vi "Get Tweets New.vi"(8 "error in":errorcluster, 9 "Tweets to Read (10)":i32=10 min=0 max=200 step=1, 10 "Screen Name (Empty)":string, 11 "Twitter Handle In":T2={"OAuth Credentials"={"Consumer Key"="", "Signature Method"=enum."HMAC-SHA1", "Token"="", "Version"="", "Token Secret"="", "Consumer Secret"=""}, "since ID"="", "max ID"="", "Screen Name"=""}) -> (0 "error out":errorcluster, 1 "Actual Num of Tweets Read":i32, 2 "New Tweets Read":T1[](array[typedef]), 3 "Twitter Handle Out":T2={"OAuth Credentials"={"Consumer Key"="", "Signature Method"=enum."HMAC-SHA1", "Token"="", "Version"="", "Token Secret"="", "Consumer Secret"=""}, "since ID"="", "max ID"="", "Screen Name"=""}, 5 "Time Stamp of Newest Tweet":timestamp)   [LabVIEW 2011, in "i3-twitter.lvlib"]
doc: "Get new tweets for the screen name. If no screen name is provided, tweets for the authenticating user are returned."
uses:
  i3-twitter.lvlib
  Controls/Twitter Handle.ctl
  i3-oauth/Controls/OAuth Credentials.ctl
  i3-oauth/Controls/Signature Method.ctl
  Controls/Tweet.ctl
  i3-oauth/Controls/HTTP Method.ctl
  i3-oauth/i3-oauth.lvlib
  <vilib>/httpClient/LabVIEWHTTPClient.lvlib
  i3-json/i3-json.lvlib
panel:
  out "headers":string
  out "body":string
  out "Full URL":string
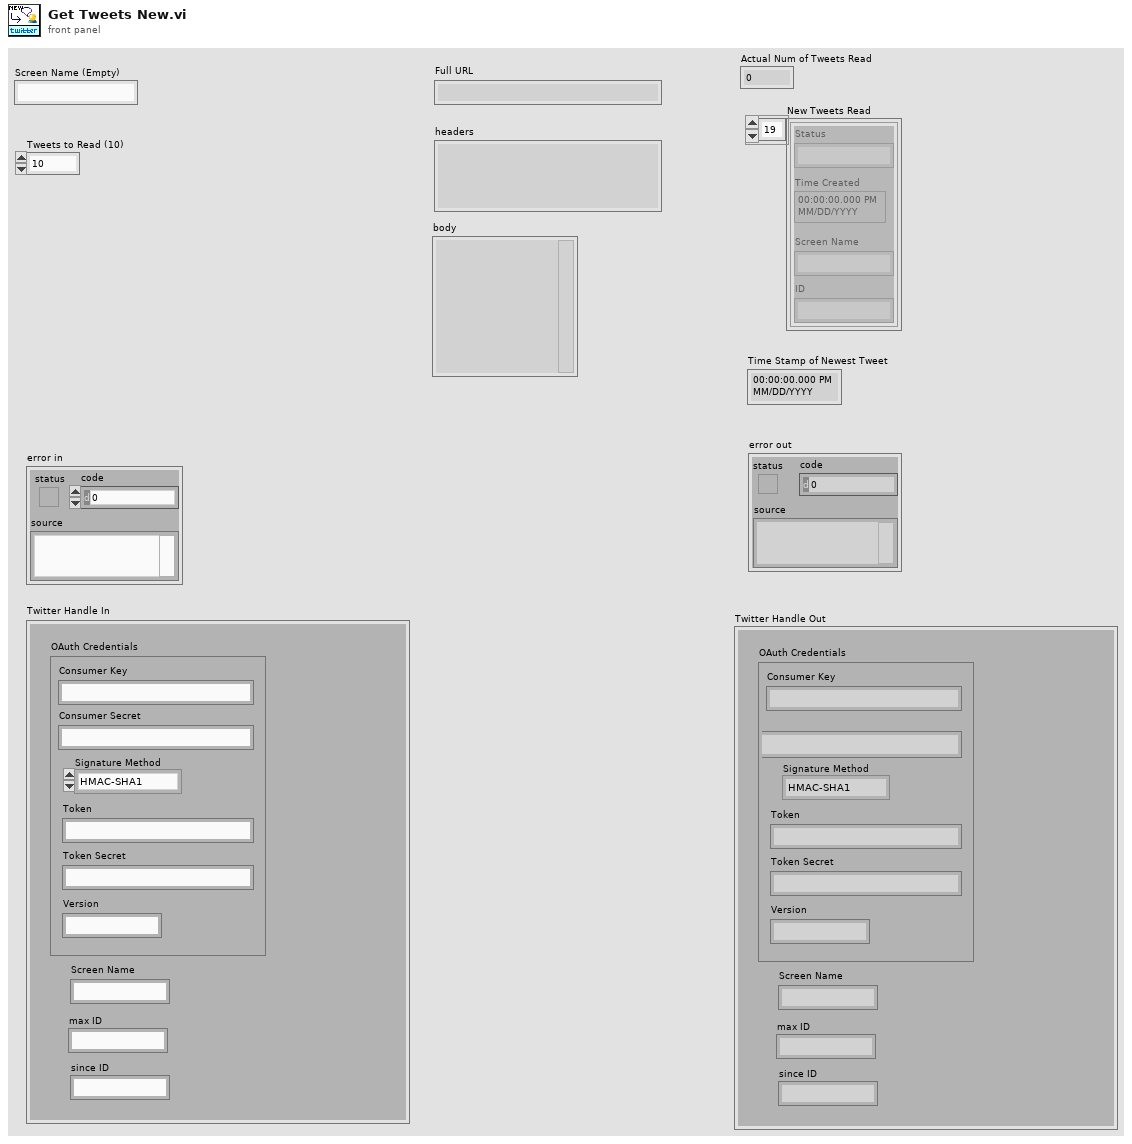
[diagram p1: front panel]
types:
  T1 = typedef "i3-twitter.lvlib/Tweet.ctl" = cluster{"Status":string, "Time Created":timestamp, "Screen Name":string, "ID":string}
  T2 = typedef "i3-twitter.lvlib/Twitter Handle.ctl" = cluster{"OAuth Credentials":T3, "since ID":string, "max ID":string, "Screen Name":string}
  T3 = typedef "i3-oauth.lvlib/OAuth Credentials.ctl" = cluster{"Consumer Key":string, "Signature Method":T4, "Token":string, "Version":string, "Token Secret":string, "Consumer Secret":string}
  T4 = typedef "i3-oauth.lvlib/Signature Method.ctl" = enum16{"HMAC-MD5", "HMAC-SHA1", "HMAC-SHA224", "HMAC-SHA256", "HMAC-SHA384", "HMAC-SHA512"}
  T5 = typedef "i3-oauth.lvlib/HTTP Method.ctl" = enum16{"GET", "POST", "PUT", "DELETE"}
  T6 = typedef "i3-oauth.lvlib/key-value-pairs.ctl" = cluster{"key":string, "value":string}
  T7 = typedef "LabVIEWHTTPClient.lvlib/ClientHandle.ctl" = refnum<k1>
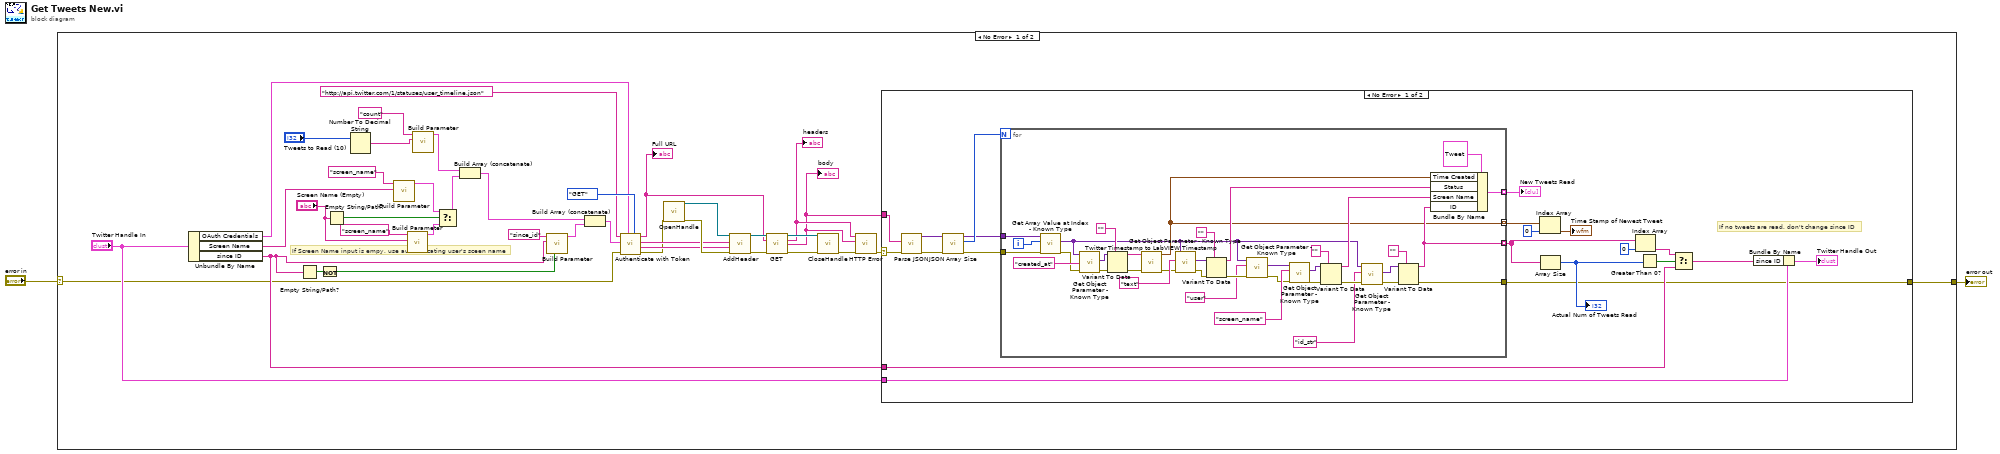
[diagram p0: block diagram]
diagram:
  n1 = case shown="No Error" "error in" {
    selector: "error in" -> [w3 w100]
    tunnel: [w8 w100] -> w2
    frame No Error {
      # "If Screen Name input is empy, use authenticating user's sceen name"
      n2 = Unbundle By Name("Twitter Handle In") -> ("OAuth Credentials"=w4:T3, "Screen Name"=w5:string, "since ID"=w6:string)
      n3 = Empty String/Path?(string/path=w6) -> (empty?=w22:bool)
      n4 = Not(x=w22) -> (.not. x?=w19:bool)
      n5 = Empty String/Path?(string/path="Screen Name (Empty)") -> (empty?=w16:bool)
      n6 = Number To Decimal String(number="Tweets to Read (10)") -> (decimal integer string=w28:string)  [unwired: 1 in]
      n7 = call "Build Parameter.vi"("Value"=w5, "Key"="screen_name") -> ("Parameter Array"=w14:T6[])  [unwired: 9 in]
      n8 = call "Build Parameter.vi"("Value"="Screen Name (Empty)", "Key"="screen_name") -> ("Parameter Array"=w13:T6[])  [unwired: 9 in]
      n9 = call "Build Parameter.vi"("Value"=w28, "Key"="count") -> ("Parameter Array"=w26:T6[])  [unwired: 9 in]
      n10 = Select(t=w14, s=w16, f=w13) -> (s? t:f=w15:T6[])
      n11 = Build Array (concatenate)(w26, w15) -> (w25:T6[])
      n12 = call "Build Parameter.vi"("Return Parameter? (T)"=w19, "Value"=w6, "Key"="since_id") -> ("Parameter Array"=w21:T6[])  [unwired: 8 in]
      n13 = Build Array (concatenate)(w25, w21) -> (w24:T6[])
      n14 = call "Authenticate with Token.vi"("HTTP Method"=HTTP_Method."GET", "OAuth Credentials"=w4, "error in (no error)"=w3, "URL Parameters"=w24, "Base URL"="http://api.twitter.com/1/statuses/user_timeline.json") -> ("error out"=w23:errorcluster, "Header Value"=w33:string, "Header Parameter"=w34:string, "Full URL"=w31:string)  [unwired: 2 in, 1 out]
      "Full URL" <- w31
      n15 = call <vilib>:"OpenHandle.vi"("error in (no error)"=w23) -> ("client handle out"=w40:T7, "error out"=w39:errorcluster)  [unwired: 13 in]
      n16 = call <vilib>:"AddHeader.vi"("client handle"=w40, "header"=w34, "value"=w33, "error in (no error)"=w39) -> ("client handle out"=w38:T7, "error out"=w37:errorcluster)  [unwired: 10 in]
      n17 = call <vilib>:"GET.vi"("client handle"=w38, "url"=w31, "error in (no error)"=w37) -> ("client handle out"=w36:T7, "headers"=w12:string, "body"=w7:string, "error out"=w35:errorcluster)  [unwired: 9 in]
      "body" <- w7
      "headers" <- w12
      n18 = call <vilib>:"CloseHandle.vi"("client handle"=w36, "error in (no error)"=w35) -> ("error out"=w11:errorcluster)  [unwired: 13 in]
      n19 = call "HTTP Error.vi"("error in (no error)"=w11, "Body"=w7, "Header"=w12) -> ("error out"=w9:errorcluster)  [unwired: 6 in, 2 out]
      n20 = case shown="No Error" w9 {
        selector: w9 -> [w48 w99]
        tunnel: w6 -> [w51 _]
        tunnel: "Twitter Handle In" -> [w50 _]
        tunnel: [w47 w99] -> w8
        tunnel: w7 -> [w46 _]
        frame No Error {
          # "If no tweets are read, don't change since ID"
          n21 = call "Parse JSON.vi"("error in (no error)"=w48, "JSON String"=w46) -> ("error out"=w59:errorcluster, "JSON Tree"=w61:variant)  [unwired: 6 in, 2 out]
          n22 = call "JSON Array Size.vi"("error in (no error)"=w59, "JSON Tree In (JSON Array)"=w61) -> ("error out"=w58:errorcluster, "Array Size"=w62:i32, "JSON Tree Passthrough (JSON Array)"=w52:variant)  [unwired: 7 in]
          n23 = for {
            N: w62 -> [_]
            tunnel: [w79] -> w60 mode=indexing
            tunnel: w58 -> [w70]
            tunnel: [w81] -> w57 mode=indexing
            tunnel: [w80] -> w47
            tunnel: w52 -> [w69]
            tunnel: [w68] -> w45 mode=indexing
            i -> [w88]
            n24 = call "Get Array Value at Index - Known Type.vi"("error in (no error)"=w70, "Index"=w88, "JSON Tree In (JSON Array)"=w69) -> ("error out"=w84:errorcluster, "Value"=w67:variant)  [unwired: 3 in, 4 out]
            n25 = call "Get Object Parameter - Known Type.vi"("error in (no error)"=w84, "Parameter Name"="created_at", "JSON Tree In (JSON Object)"=w67) -> ("error out"=w78:errorcluster, "Value"=w76:variant)  [unwired: 3 in, 4 out]
            n26 = Variant To Data(error in=w78, type="", Variant=w76) -> (data=w87:string, error out=w74:errorcluster)
            n27 = call "Twitter Timestamp to LabVIEW Timestamp.vi"("error in"=w74, "Twitter Time Stamp"=w87) -> ("error out"=w73:errorcluster, "LabVIEW Time Stamp"=w68:timestamp)  [unwired: 6 in]
            n28 = call "Get Object Parameter - Known Type.vi"("error in (no error)"=w73, "Parameter Name"="text", "JSON Tree In (JSON Object)"=w67) -> ("error out"=w77:errorcluster, "Value"=w96:variant)  [unwired: 3 in, 4 out]
            n29 = Variant To Data(error in=w77, type="", Variant=w96) -> (data=w71:string, error out=w75:errorcluster)
            n30 = call "Get Object Parameter - Known Type.vi"("error in (no error)"=w75, "Parameter Name"="user", "JSON Tree In (JSON Object)"=w67) -> ("error out"=w83:errorcluster, "Value"=w66:variant)  [unwired: 3 in, 4 out]
            n31 = call "Get Object Parameter - Known Type.vi"("error in (no error)"=w83, "Parameter Name"="screen_name", "JSON Tree In (JSON Object)"=w66) -> ("error out"=w82:errorcluster, "Value"=w92:variant)  [unwired: 3 in, 4 out]
            n32 = Variant To Data(error in=w82, type="", Variant=w92) -> (data=w93:string, error out=w72:errorcluster)
            n33 = call "Get Object Parameter - Known Type.vi"("error in (no error)"=w72, "Parameter Name"="id_str", "JSON Tree In (JSON Object)"=w67) -> ("error out"=w86:errorcluster, "Value"=w65:variant)  [unwired: 3 in, 4 out]
            n34 = Variant To Data(error in=w86, type="", Variant=w65) -> (data=w79:string, error out=w80:errorcluster)
            n35 = Bundle By Name(cluster=T1 {"Status"="", "Time Created"=timestamp(0 s since 1904-01-01), "Screen Name"="", "ID"=""}, "Time Created"=w68, "Status"=w71, "Screen Name"=w93, "ID"=w79) -> (w81:T1)
          }
          "New Tweets Read" <- w57
          n36 = Index Array(array=w45, index=0) -> (element=→"Time Stamp of Newest Tweet":timestamp)
          n37 = Array Size(array=w60) -> (size(s)=w55:i32)
          "Actual Num of Tweets Read" <- w55
          n38 = Index Array(array=w60, index=0) -> (element=w54:string)
          n39 = Greater Than 0?(x=w55) -> (x > 0?=w56:bool)
          n40 = Select(t=w54, s=w56, f=w51) -> (s? t:f=w53:string)
          n41 = Bundle By Name(cluster=w50, "since ID"=w53) -> (→"Twitter Handle Out":T2)
        }
        frame Error {
        }
      }
    }
    frame Error {
    }
  }
  "error out" <- w2
